vi "Read DriverXBoxController.vi"(8 "error in (no error)":errorcluster, 11 "DriverStation in":refnum<class "DriverStation.lvclass">) -> (0 "error out":errorcluster, 2 "XBoxController":refnum<class "XBoxController.lvclass">, 3 "DriverStation out":refnum<class "DriverStation.lvclass">)   [LabVIEW 2013, in "DriverStation.lvclass"]
uses:
  DriverStation.lvclass
  XboxController/XBoxController.lvclass
  DriverStation.lvclass/DriverStation.ctl
  DriverXBoxController/DriverXBoxController.lvclass
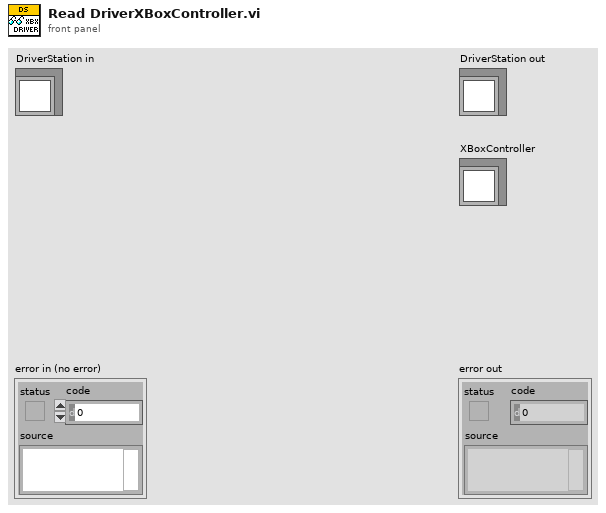
[diagram p1: front panel]
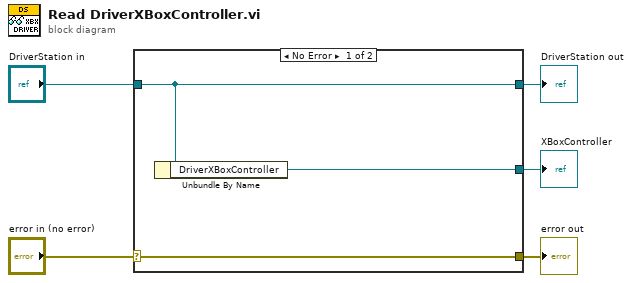
[diagram p0: block diagram]
diagram:
  n1 = case shown="No Error" "error in (no error)" {
    selector: "error in (no error)" -> [w8 w9]
    tunnel: [w8 w9] -> w4
    tunnel: [w7 w10] -> w2
    tunnel: "DriverStation in" -> [w7 w10]
    tunnel: [w6 _] -> w1
    frame No Error {
      n2 = Unbundle By Name(w7) -> ("DriverXBoxController"=w6:refnum<class "DriverXBoxController.lvclass">)
    }
    frame Error {
    }
  }
  "error out" <- w4
  "DriverStation out" <- w2
  "XBoxController" <- w1
